vi "Get Sorted Streams.vi"(8 "error in (no error)":errorcluster, 11 "PXImc Transceiver in":refnum<class "DSF PXImc Transceiver.lvclass">=refnum) -> (0 "error out":errorcluster, 2 "stream-sorted transfers":T1[](array[typedef]), 3 "PXImc Transceiver out":refnum<class "DSF PXImc Transceiver.lvclass">)   [LabVIEW 2017, in "DSF Core.lvlib" / "DSF PXImc Transceiver.lvclass"]
uses:
  DSF PXImc Transceiver.lvclass
  PXImc Transfer Data.ctl
  DSF PXImc Transceiver.lvclass/DSF PXImc Transceiver.ctl
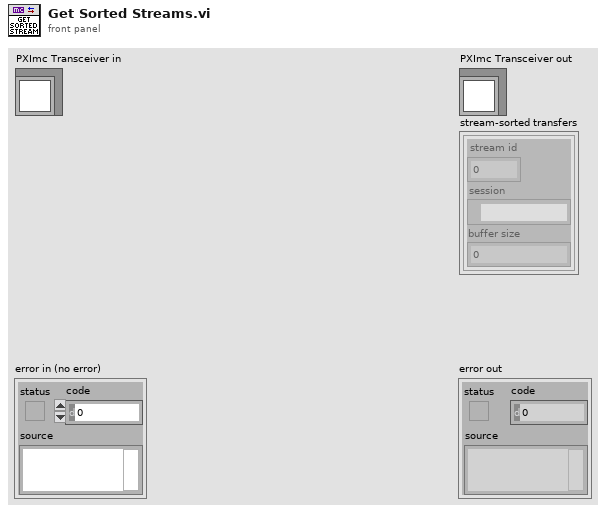
[diagram p1: front panel]
types:
  T1 = typedef "DSF Core.lvlib/DSF PXImc Transceiver.lvclass/PXImc Transfer Data.ctl" = cluster{"stream id":u16, "session":refnum<k21>, "buffer size":u64}
  T2 = typedef "DSF Core.lvlib/DSF PXImc Transceiver.lvclass/PXImc Group Data.ctl" = cluster{"direction":T3, "transfers":T1[]}
  T3 = typedef "DSF Core.lvlib/DSF Direction.ctl" = enum8{"Tx", "Rx"}
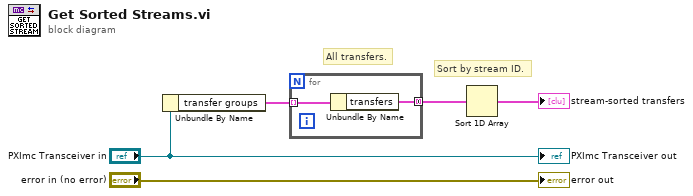
[diagram p0: block diagram]
diagram:
  # "All transfers."
  # "Sort by stream ID."
  n1 = Unbundle By Name("PXImc Transceiver in") -> ("transfer groups"=w4:T2[])
  n2 = for {
    tunnel: w4 -> [w7] mode=indexing
    tunnel: [w6] -> w5 mode=concatenating
    n3 = Unbundle By Name(w7) -> ("transfers"=w6:T1[])
  }
  n4 = Sort 1D Array(array=w5) -> (sorted array=→"stream-sorted transfers":T1[])
  "error out" <- "error in (no error)"
  "PXImc Transceiver out" <- "PXImc Transceiver in"
